vi "Scale Air Flow.vi"(7 "Run Mode":T1, 10 "Air Flow (cfm)":dbl) -> (1 "Air Flow (cfm) out":dbl, 2 "Air Voltage out":dbl)   [LabVIEW 2013]
doc: "This sub-VI scales desired air flow in cubic-feet-per-minute to the appropriate voltage needed to control\nthe parallel air valves that control the air flow."
uses:
  Controls/run_mode_enum.ctl
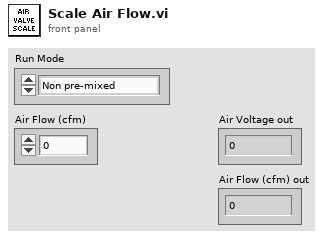
[diagram p1: front panel]
types:
  T1 = typedef "run_mode_enum.ctl" = enum16{"Non pre-mixed", "Pre-mixed"}
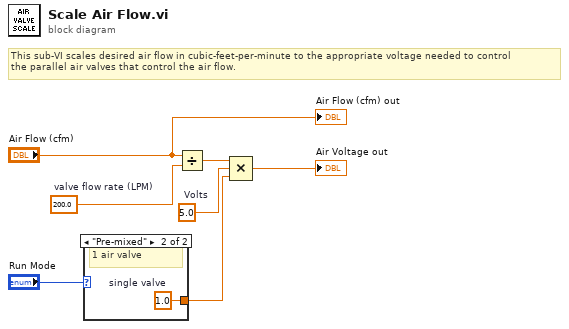
[diagram p0: block diagram]
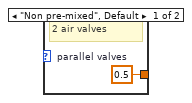
[diagram p2: hidden frame]
diagram:
  w3 = 5.0  # Volts
  w6 = 200.0  # valve flow rate (LPM)
  # "This sub-VI scales desired air flow in cubic-feet-per-minute to the appropriate voltage needed to control\nthe parallel air valves that control the air flow."
  n1 = case shown="\"Pre-mixed\"" "Run Mode" {
    tunnel: [w8 w9] -> w1
    frame "Non pre-mixed", Default {
      w8 = 0.5  # parallel valves
      # "2 air valves"
    }
    frame "Pre-mixed" {
      w9 = 1.0  # single valve
      # "1 air valve"
    }
  }
  n2 = Divide(x="Air Flow (cfm)", y=w6) -> (x/y=w4:dbl)
  n3 = Compound Arithmetic op=MULTIPLY(w4, w3, w1) -> (→"Air Voltage out":dbl)
  "Air Flow (cfm) out" <- "Air Flow (cfm)"
